vi "commandA.vi"() -> ()   [LabVIEW 2013]
panel:
  in  "element":u8
  in  "K":u8
  out "output array":u8[](array[numeric])
  out "Bit Sync":u8[](array[numeric])
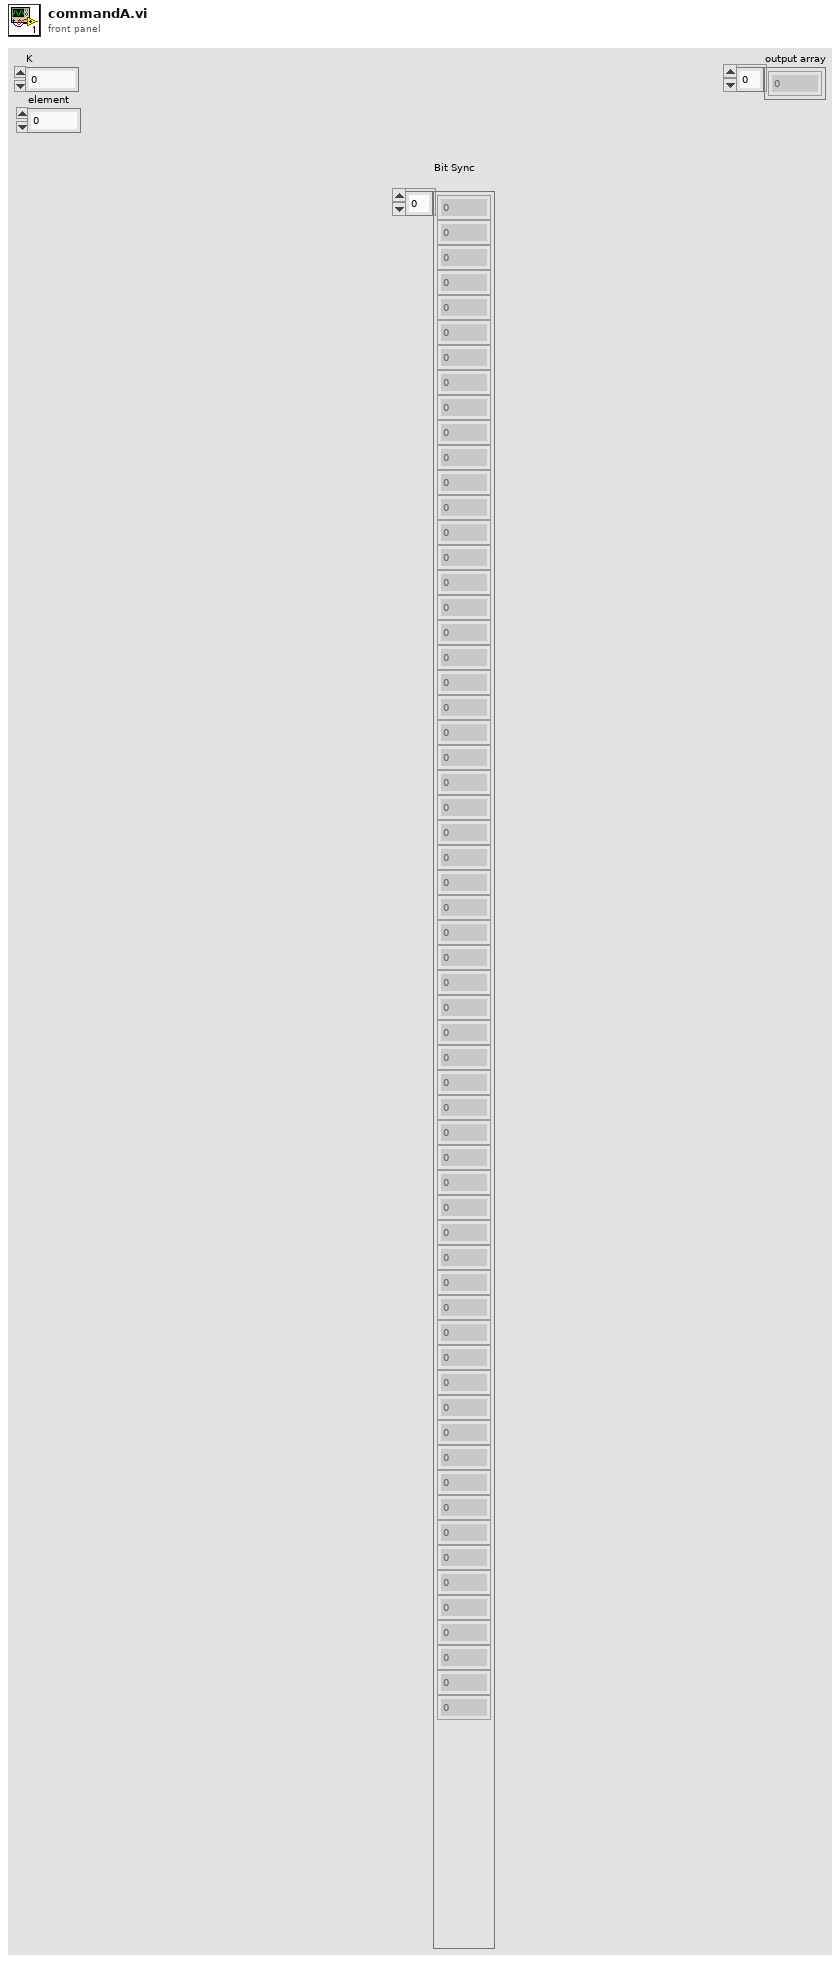
[diagram p1: front panel]
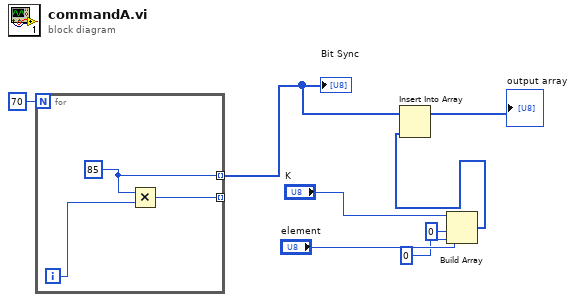
[diagram p0: block diagram]
diagram:
  n1 = for {
    N: 70 -> [_]
    tunnel: [w10] -> _ mode=indexing
    tunnel: [w9] -> w7 mode=indexing
    i -> [w11]
    w9 = u8 85 ("x")
    n2 = Multiply(x=w9, y=w11) -> (x*y=w10:i32)
  }
  "Bit Sync" <- w7
  n3 = Build Array("K", "element", u8 0 ("element"), u8 0 ("element")) -> (w2:u8[])
  n4 = Insert Into Array(array=w7, new element=w2) -> (→"output array":u8[])  [unwired: 1 in]
